vi "Conf Current.vi"(0 "VISA Resource Name":refnum<visa-resource-name>, 1 "Check/Set (F:Set)":bool, 2 "Check Parameter(1:Ap Min)":T3(ring)=enum."Aperture Min", 5 "AC/DC (F:DC)":bool, 7 "Autorange On? (F:Off)":bool, 9 "Range (4:Maximum)":T2(ring)=enum."Maximum", 11 "error in (no error)":errorcluster, 12 "Channel List (empty)":string, 13 "Advanced Config":T1={"Aperture Value (.4)"=0.4, "Aperture (1:Minimum)"=1, "NPLC (1)"=2, "Bandwidth (3 Hz)"=0, "Integration Time (F:Aperture)"=FALSE} {"Bandwidth (3 Hz)" items=["3", "20", "200", "MIN", "MAX"]; "NPLC (1)" items=[".02", ".2", "1", "2", "10", "20", "100", "200", "Minimum", "Maximum"]; "Aperture (1:Minimum)" items=["Manual", "Minimum", "Maximum"]; "Aperture Value (.4)" min=0.4 max=4.0 format="%.2f"}) -> (4 "VISA Resource Name Out":refnum<visa-resource-name>, 8 "Configuration?":string, 15 "error out":errorcluster)   [LabVIEW 2012, in "Agilent 34970.lvlib"]
doc: "This VI configures the instrument for advanced current measurements. This VI is only valid for channels 21 and 22 on the 39401 A module.\n\nThis is an advanced measurment configuration VI. For more information on the different ways to take and configure a measurment, refer to the context help and block diagram of \"HP34970A Advanced Scan Example.vi\"."
uses:
  <instrlib>/Agilent 34970/Agilent 34970.lvlib
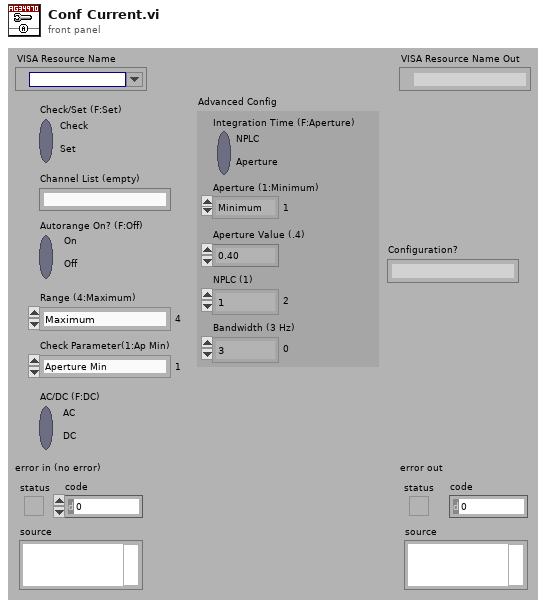
[diagram p1: front panel]
types:
  T1 = cluster{"Aperture Value (.4)":dbl, "Aperture (1:Minimum)":u16, "NPLC (1)":u16, "Bandwidth (3 Hz)":u16, "Integration Time (F:Aperture)":bool}
  T2 = enum16{"10 mA", "100 mA", "1 A", "Minimum", "Maximum"}
  T3 = enum16{"Aperture (By Chan)", "Aperture Min", "Aperture Max", "NPLC (By Chan)", "NPLC Min", "NPLC Max", "Bandwidth (By Chan)", "Bandwidth Min", "Bandwidth Max"}
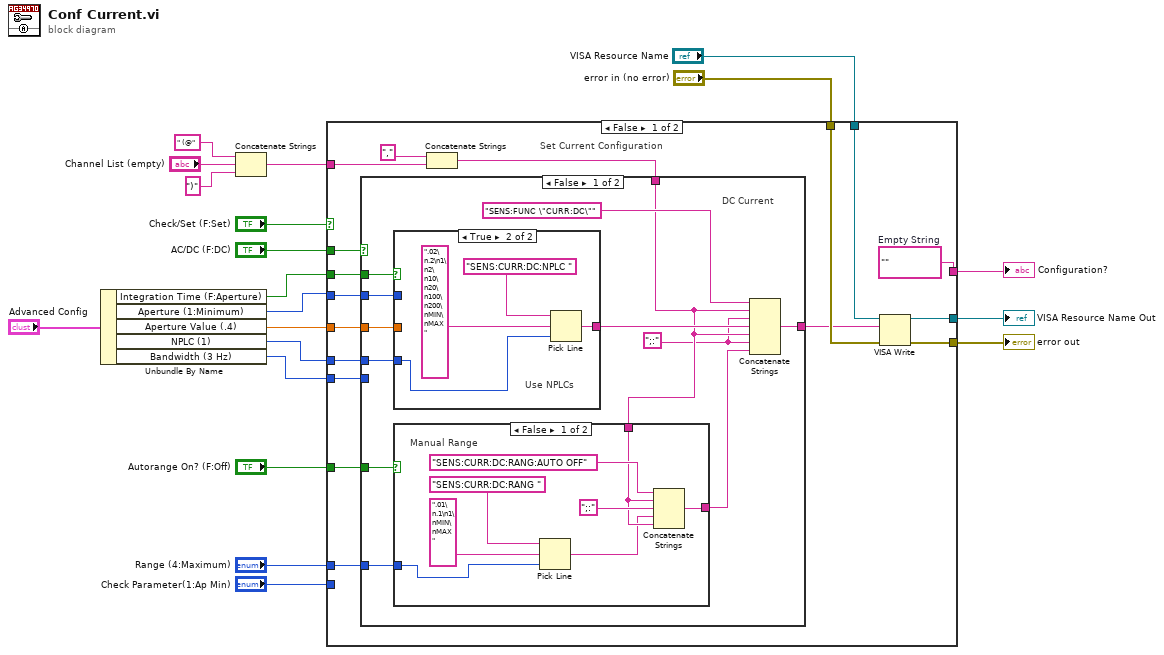
[diagram p0: block diagram]
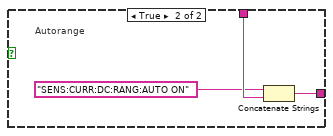
[diagram p2: hidden frame]
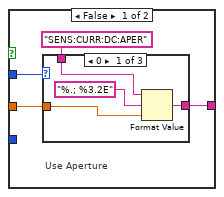
[diagram p3: hidden frame]
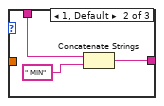
[diagram p4: hidden frame]
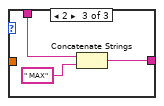
[diagram p5: hidden frame]
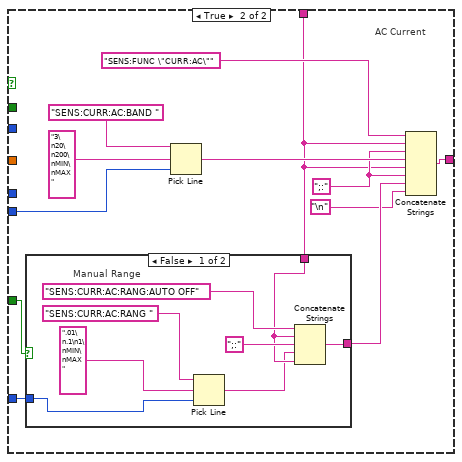
[diagram p6: hidden frame]
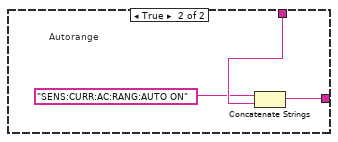
[diagram p7: hidden frame]
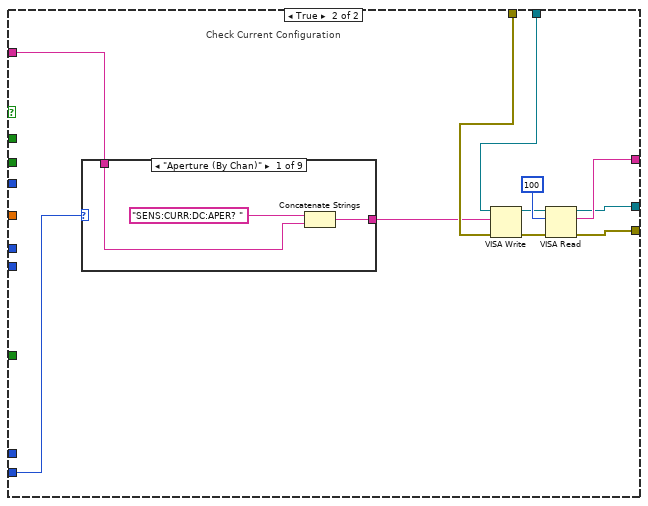
[diagram p8: hidden frame]
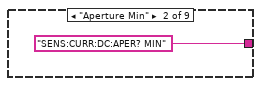
[diagram p9: hidden frame]
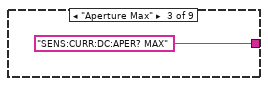
[diagram p10: hidden frame]
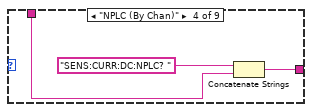
[diagram p11: hidden frame]
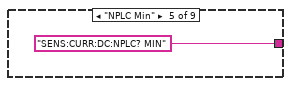
[diagram p12: hidden frame]
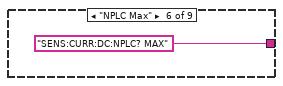
[diagram p13: hidden frame]
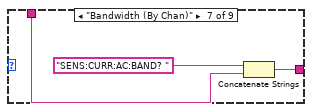
[diagram p14: hidden frame]
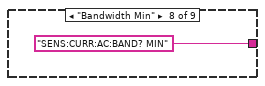
[diagram p15: hidden frame]
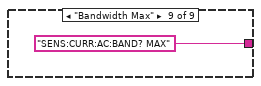
[diagram p16: hidden frame]
diagram:
  n1 = Unbundle By Name("Advanced Config") -> ("Integration Time (F:Aperture)"=w12:bool, "Aperture (1:Minimum)"=w11:u16, "Aperture Value (.4)"=w10:dbl, "NPLC (1)"=w9:u16, "Bandwidth (3 Hz)"=w8:u16)
  n2 = Concatenate Strings(" (@", "Channel List (empty)", ")") -> (w15:string)
  n3 = case shown="False" "Check/Set (F:Set)" {
    tunnel: [w27 w112] -> w4
    tunnel: "AC/DC (F:DC)" -> [w37 _]
    tunnel: w11 -> [w36 _]
    tunnel: w10 -> [w35 _]
    tunnel: w9 -> [w34 _]
    tunnel: w15 -> [w33 w105]
    tunnel: w8 -> [w30 _]
    tunnel: [w29 w110] -> w14
    tunnel: "error in (no error)" -> [w28 w109]
    tunnel: "Check Parameter(1:Ap Min)" -> [_ w106]
    tunnel: w12 -> [w26 _]
    tunnel: "Autorange On? (F:Off)" -> [w24 _]
    tunnel: "Range (4:Maximum)" -> [w23 _]
    tunnel: [w22 w104] -> w3
    tunnel: "VISA Resource Name" -> [w21 w103]
    frame False {
      w29 = ""  # Empty String
      # "Set Current Configuration"
      n4 = Concatenate Strings(",", w33) -> (w31:string)
      n5 = case shown="False" w37 {
        tunnel: w36 -> [w45 _]
        tunnel: w35 -> [w46 _]
        tunnel: w34 -> [w44 _]
        tunnel: w31 -> [w40 w80]
        tunnel: w30 -> [_ w87]
        tunnel: [w48 w86] -> w25
        tunnel: w26 -> [w47 _]
        tunnel: w24 -> [w42 w83]
        tunnel: w23 -> [w41 w84]
        frame False {
          w39 = ";:"
          # "DC Current"
          n6 = case shown="True" w47 {
            tunnel: w46 -> [w63 _]
            tunnel: w45 -> [w62 _]
            tunnel: w44 -> [_ w76]
            tunnel: [w61 w75] -> w43
            frame False {
              # "Use Aperture"
              n7 = case shown="0" w62 {
                tunnel: "SENS:CURR:DC:APER" -> [w68 w71 w73]
                tunnel: [w66 w69 w72] -> w61
                tunnel: w63 -> [w65 _ _]
                frame 0 {
                  n8 = Format Value(string ("")=w68, format string="%.; %3.2E", value (0)=w65) -> (output string=w66:string)
                }
                frame 1, Default {
                  n9 = Concatenate Strings(w71, " MIN") -> (w69:string)
                }
                frame 2 {
                  n10 = Concatenate Strings(w73, " MAX") -> (w72:string)
                }
              }
            }
            frame True {
              # "Use NPLCs"
              n11 = Pick Line(string ("")="SENS:CURR:DC:NPLC ", multi-line string=".02\n.2\n1\n2\n10\n20\n100\n200\nMIN\nMAX", line index=w76) -> (output string=w75:string)
            }
          }
          n12 = case shown="False" w42 {
            tunnel: w41 -> [w50 _]
            tunnel: w40 -> [w53 w60]
            tunnel: [w52 w58] -> w38
            frame False {
              # "Manual Range"
              n13 = Pick Line(string ("")="SENS:CURR:DC:RANG ", multi-line string=".01\n.1\n1\nMIN\nMAX", line index=w50) -> (output string=w51:string)
              n14 = Concatenate Strings("SENS:CURR:DC:RANG:AUTO OFF", w53, ";:", w51, w53) -> (w52:string)
            }
            frame True {
              # "Autorange"
              n15 = Concatenate Strings("SENS:CURR:DC:RANG:AUTO ON", w60) -> (w58:string)
            }
          }
          n16 = Concatenate Strings("SENS:FUNC \"CURR:DC\"", w40, w39, w43, w40, w39, w38) -> (w48:string)
        }
        frame True {
          w82 = ";:"
          # "AC Current"
          n17 = case shown="False" w83 {
            tunnel: w84 -> [w96 _]
            tunnel: w80 -> [w93 w101]
            tunnel: [w92 w99] -> w81
            frame False {
              # "Manual Range"
              n18 = Pick Line(string ("")="SENS:CURR:AC:RANG ", multi-line string=".01\n.1\n1\nMIN\nMAX", line index=w96) -> (output string=w91:string)
              n19 = Concatenate Strings("SENS:CURR:AC:RANG:AUTO OFF", w93, ";:", w91, w93) -> (w92:string)
            }
            frame True {
              # "Autorange"
              n20 = Concatenate Strings("SENS:CURR:AC:RANG:AUTO ON", w101) -> (w99:string)
            }
          }
          n21 = Pick Line(string ("")="SENS:CURR:AC:BAND ", multi-line string="3\n20\n200\nMIN\nMAX", line index=w87) -> (output string=w88:string)
          n22 = Concatenate Strings("SENS:FUNC \"CURR:AC\"", w80, w82, w88, w80, w82, w81, "\n" ("Line Feed Constant")) -> (w86:string)
        }
      }
      n23 = VISA Write(VISA resource name=w21, write buffer=w25, error in (no error)=w28) -> (VISA resource name out=w22:refnum<visa-resource-name>, error out=w27:errorcluster)  [unwired: 1 out]
    }
    frame True {
      # "Check Current Configuration"
      n24 = case shown="\"Aperture (By Chan)\"" w106 {
        tunnel: w105 -> [w115 _ _ w119 _ _ w124 _ _]
        tunnel: [w113 "SENS:CURR:DC:APER? MIN" "SENS:CURR:DC:APER? MAX" w118 "SENS:CURR:DC:NPLC? MIN" "SENS:CURR:DC:NPLC? MAX" w123 "SENS:CURR:AC:BAND? MIN" "SENS:CURR:AC:BAND? MAX"] -> w102
        frame "Aperture (By Chan)" {
          n25 = Concatenate Strings("SENS:CURR:DC:APER? ", w115) -> (w113:string)
        }
        frame "Aperture Min" {
        }
        frame "Aperture Max" {
        }
        frame "NPLC (By Chan)" {
          n26 = Concatenate Strings("SENS:CURR:DC:NPLC? ", w119) -> (w118:string)
        }
        frame "NPLC Min" {
        }
        frame "NPLC Max" {
        }
        frame "Bandwidth (By Chan)" {
          n27 = Concatenate Strings("SENS:CURR:AC:BAND? ", w124) -> (w123:string)
        }
        frame "Bandwidth Min" {
        }
        frame "Bandwidth Max" {
        }
      }
      n28 = VISA Write(VISA resource name=w103, write buffer=w102, error in (no error)=w109) -> (VISA resource name out=w108:refnum<visa-resource-name>, error out=w107:errorcluster)  [unwired: 1 out]
      n29 = VISA Read(VISA resource name=w108, byte count=u32 100 ("byte count (0)"), error in (no error)=w107) -> (VISA resource name out=w104:refnum<visa-resource-name>, read buffer=w110:string, error out=w112:errorcluster)  [unwired: 1 out]
    }
  }
  "Configuration?" <- w14
  "error out" <- w4
  "VISA Resource Name Out" <- w3
